vi "Main.vi"(11 "Module Admin":refnum<class "Delacor_lib_QMH_Module Admin.lvclass">) -> ()   [LabVIEW 2019, in "Acquisition.lvlib"]
doc: "This template is based off of the Queued Message Handler design pattern and the Queued Message Handler project template that ships with LabVIEW.\n\nThe main difference is that the queue is private to this module and communication between modules is performed via Broadcast and Request events.\n\nRequest events are wrapped in public API methods and are handled in the Event Handling Loop (EHL) of this VI. Any module can register for Broadcast events sent by this module. The EHL generates messages based on user interface actions.\n\nThe Message Handling Loop (MHL) processes messages generated by the EHL, or by other messages. The messages are string values, so new messages can be added easily to the Message Cases case structure in the MHL. Each message cluster can also provide an optional value for Message Data, which is a variant that can be converted to whatever message-specific data is required.\n_____\nBased on Delacor QMH Project Template 5.0.0.82."
uses:
  Acquisition.lvlib
  <vilib>/Delacor/Delacor QMH/Libraries/Module Admin_class/Delacor_lib_QMH_Module Admin.lvclass
  Module Data--cluster.ctl
  Stop Helper Loop Argument--cluster.ctl
  Stop Argument--cluster.ctl
  <vilib>/Delacor/Delacor QMH/Libraries/Message Queue_class/Delacor_lib_QMH_Message Queue.lvclass/Delacor_lib_QMH_Message Queue.ctl
  <vilib>/Delacor/Delacor QMH/Libraries/Module Admin_class/Delacor_lib_QMH_Module Admin.lvclass/Delacor_lib_QMH_Module Admin.ctl
  Start Aquire Argument--cluster.ctl
  Stop Acquire Argument--cluster.ctl
  <vilib>/Utility/miscctls.llb/LVPointTypeDef.ctl
  <vilib>/Delacor/Delacor QMH/Libraries/Message Queue_class/Delacor_lib_QMH_Enqueue Message (Single).vi
  <vilib>/Delacor/Delacor QMH/Libraries/Module Admin_class/Delacor_lib_QMH_Get External Launch.vi
  <vilib>/Utility/error.llb/Error Cluster From Error Code.vi
  <vilib>/ErrorRing/Error Ring.xnode
  <vilib>/Delacor/Delacor QMH/Libraries/Message Queue_class/Delacor_lib_QMH_Message Queue.lvclass
panel:
  out "Waveform Graph - Dark":dynamicdata(graph)
  out "error out":errorcluster
  out "Status":string
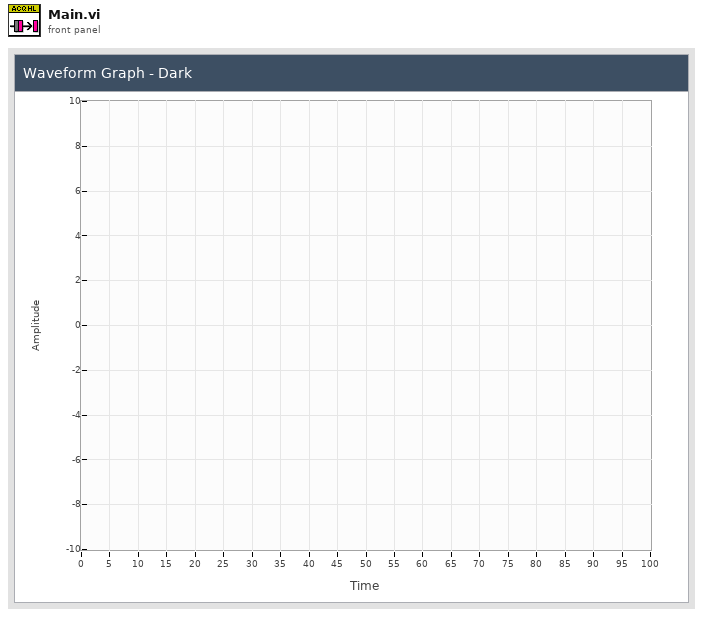
[diagram p1: front panel]
types:
  T1 = typedef "Acquisition.lvlib/Request Events--cluster.ctl" = cluster{"Stop Module":refnum<user-event>, "Show Panel":refnum<user-event>, "Hide Panel":refnum<user-event>, "Get Module Execution Status":refnum<user-event>, "Show Diagram":refnum<user-event>, "Start Helper Loop":refnum<user-event>, "Stop Helper Loop":refnum<user-event>, "Start Aquire":refnum<user-event>, "Stop Acquire":refnum<user-event>}
  T2 = typedef "Acquisition.lvlib/Module Data--cluster.ctl" = cluster{"Status":string}
  T3 = typedef "Acquisition.lvlib/Stop Helper Loop Argument--cluster.ctl" = cluster{"Boolean":bool}
  T4 = enum32{"invalid lock state", "Not Locked", "Locked (No Password)", "Password-protected"}
  T5 = typedef "Acquisition.lvlib/Stop Argument--cluster.ctl" = cluster{"Origin":string, "Exit via Stop Module Req?":bool, "Wait for Module to stop?":bool}
  T6 = typedef "Acquisition.lvlib/Start Aquire Argument--cluster.ctl" = cluster{"Boolean":bool}
  T7 = typedef "Acquisition.lvlib/Stop Acquire Argument--cluster.ctl" = cluster{"Boolean":bool}
  T8 = typedef "LVPointTypeDef.ctl" = cluster{"Horizontal":i16, "Vertical":i16}
  T9 = enum32{"Invalid", "Standard", "Closed", "Hidden", "Minimized", "Maximized"}
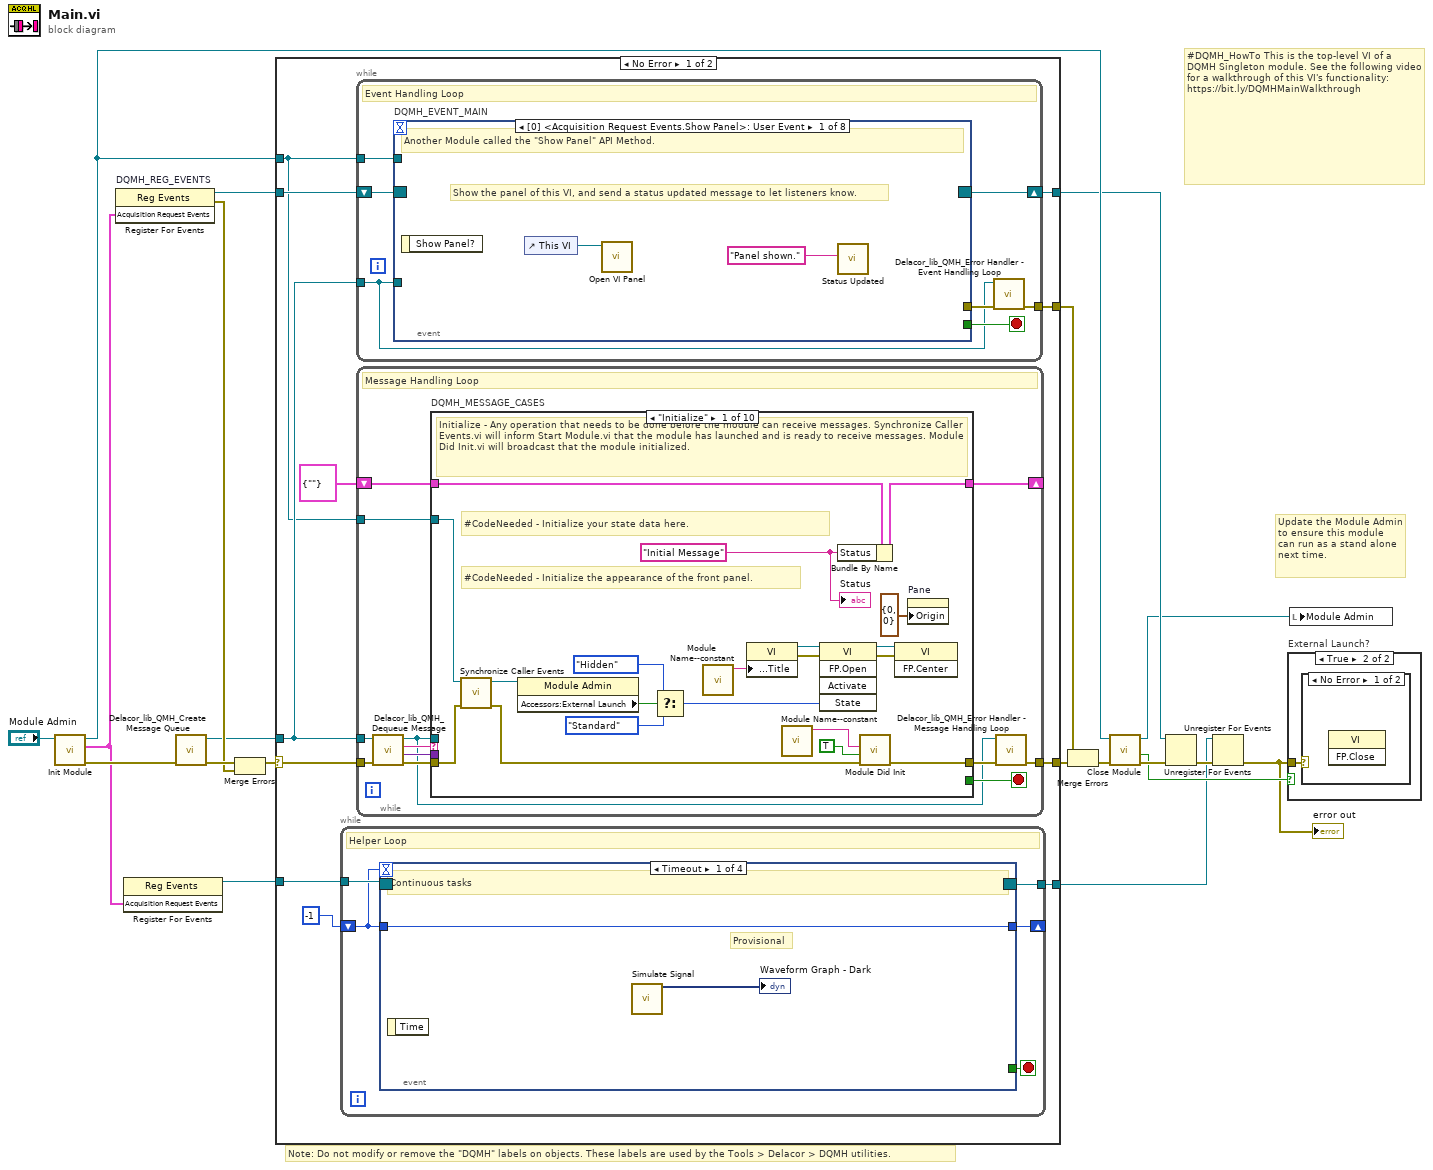
[diagram p0: block diagram]
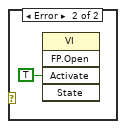
[diagram p3: hidden frame]
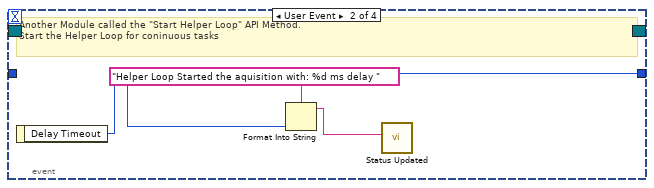
[diagram p4: hidden frame]
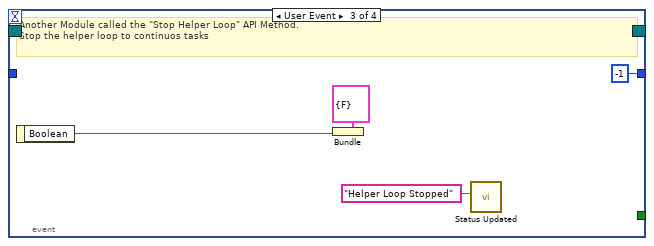
[diagram p5: hidden frame]
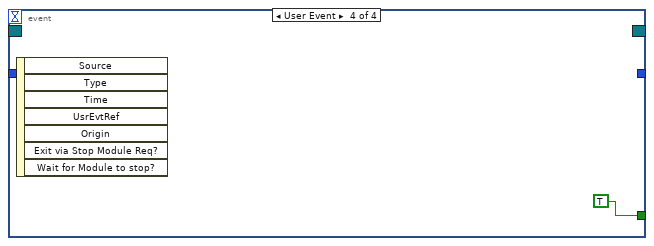
[diagram p6: hidden frame]
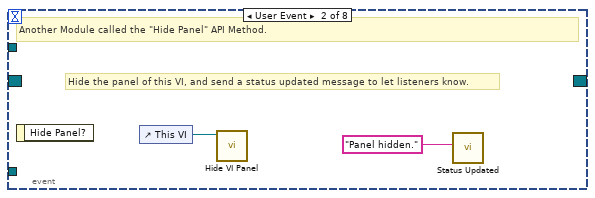
[diagram p7: hidden frame]
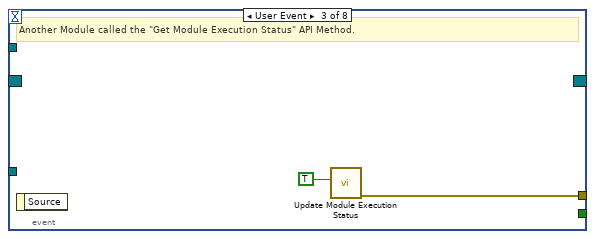
[diagram p8: hidden frame]
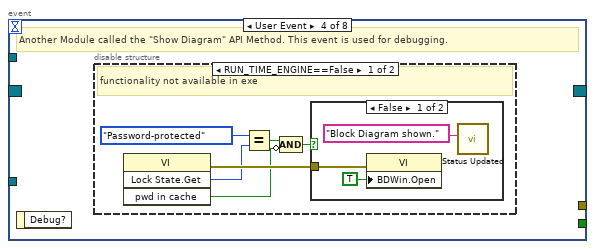
[diagram p9: hidden frame]
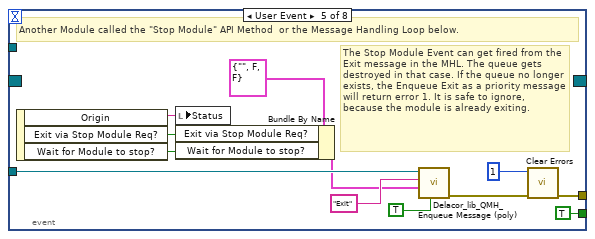
[diagram p12: hidden frame]
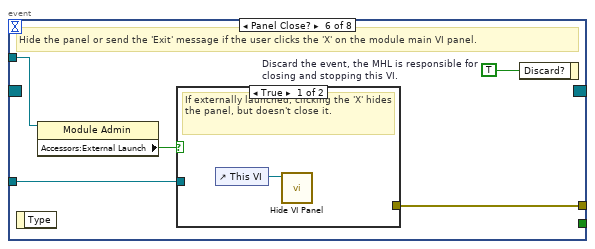
[diagram p13: hidden frame]
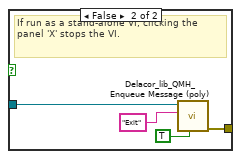
[diagram p14: hidden frame]
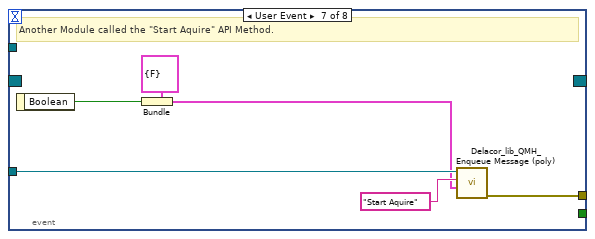
[diagram p15: hidden frame]
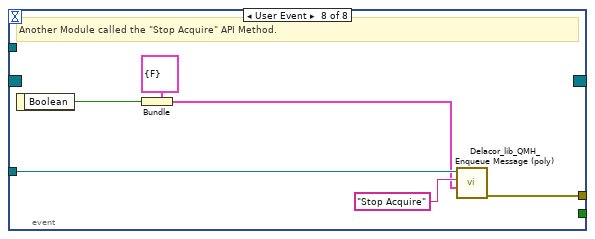
[diagram p16: hidden frame]
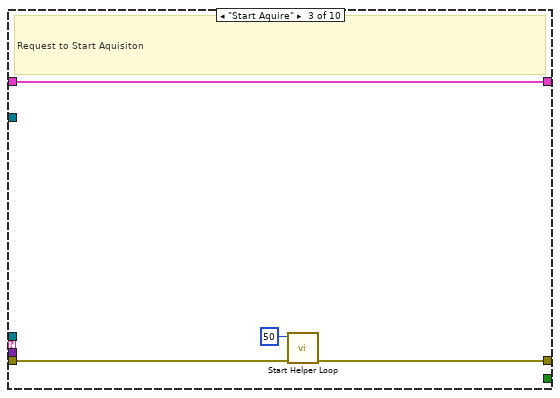
[diagram p18: hidden frame]
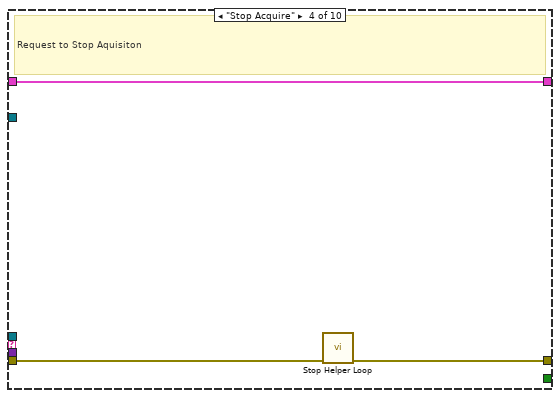
[diagram p19: hidden frame]
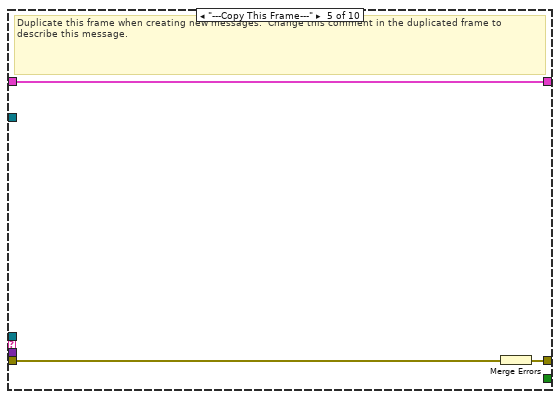
[diagram p20: hidden frame]
diagram:
  # "#DQMH_HowTo This is the top-level VI of a DQMH Singleton module. See the following video for a walkthrough of this VI's functionality: https://bit.ly/DQMHMainWalkthrough"
  # "Note: Do not modify or remove the \"DQMH\" labels on objects. These labels are used by the Tools > Delacor > DQMH utilities."
  # "Update the Module Admin to ensure this module can run as a stand alone next time."
  n1 = call "Init Module.vi"("Singleton Module Admin in"="Module Admin") -> ("error out"=w19:errorcluster, "Acquisition Request Events"=w4:T1, "Singleton Module Admin out"=w12:refnum<class "Delacor_lib_QMH_Module Admin.lvclass">)  [unwired: 8 in]
  n2 = register-events "DQMH_REG_EVENTS"(w4) -> (reference out=w10:refnum<event-registration>, error out=w13:errorcluster)  [unwired: 2 in]
  n3 = register-events(w4) -> (reference out=w5:refnum<event-registration>)  [unwired: 2 in, 1 out]
  n4 = call <vilib>:"Delacor_lib_QMH_Create Message Queue.vi"("error in (no error)"=w19) -> ("error out"=w15:errorcluster, "Message Queue"=w9:refnum<class "Delacor_lib_QMH_Message Queue.lvclass">)  [unwired: 9 in]
  n5 = Merge Errors(w15, w13) -> (w14:errorcluster)
  n6 = case shown="No Error" w14 {
    selector: w14 -> [w29 w210]
    tunnel: [w31 w209] -> w20
    tunnel: [w28 w215] -> w11
    tunnel: w10 -> [w26 w215]
    tunnel: w9 -> [w25 w208]
    tunnel: [w30 _] -> w17
    tunnel: w12 -> [w24 w211]
    tunnel: w5 -> [w23 w207]
    tunnel: [w22 w207] -> w1
    frame No Error {
      n7 = while {
        tunnel: w23 -> [w36]
        tunnel: [w35] -> w22
        shift-right: [w33] -> _
        shift-left: -1 -> [w32]
        stop <- w34 stop-if-true
        # "Helper Loop"
        n8 = event shown="[0] Timeout" {
          selector: w36 -> [_ _ _ _]
          dyn-events: [_ _ _ _] -> w35
          timeout: w32 -> [_ _ _ _]
          tunnel: [_ _ _ TRUE] -> w34
          tunnel: [w38 w41 -1 _] -> w33
          tunnel: w32 -> [w38 _ _ _]
          event Timeout {
            # "Provisional"
            # "Continuous tasks"
            n9 = event-data() -> ()  [unwired: 1 in, 1 out]
            n10 = call "Simulate Signal"() -> ("Sine"=→"Waveform Graph - Dark":dynamicdata)  [unwired: 14 in, 1 out]
          }
          event User Event {
            # "Another Module called the \"Start Helper Loop\" API Method.\nStart the Helper Loop for coninuous tasks"
            n11 = event-data() -> ("Delay Timeout"=w41:u32)  [unwired: 1 in]
            n12 = Format Into String(format string="Helper Loop Started the aquisition with: %d ms delay ", w41) -> (resulting string=w40:string)  [unwired: 2 in, 1 out]
            n13 = call "Status Updated.vi"("Status"=w40) -> ()  [unwired: 10 in, 1 out]
          }
          event User Event {
            # "Another Module called the \"Stop Helper Loop\" API Method.\nStop the helper loop to continuos tasks"
            n14 = event-data() -> ("Boolean"=w44:bool)  [unwired: 1 in]
            n15 = Bundle(cluster=T3 {"Boolean"=FALSE} ("Stop Helper Loop Argument"), "Boolean"=w44) -> ()  [unwired: 1 out]
            n16 = call "Status Updated.vi"("Status"="Helper Loop Stopped") -> ()  [unwired: 10 in, 1 out]
          }
          event User Event {
            n17 = event-data() -> ()  [unwired: 1 in, 7 out]
          }
        }
      }
      n18 = while {
        tunnel: w25 -> [w47]
        shift-right: [w50] -> w28
        shift-left: w26 -> [w51]
        tunnel: [w52] -> w30
        tunnel: w24 -> [w48]
        stop <- w49 stop-if-true
        # "Event Handling Loop"
        n19 = event "DQMH_EVENT_MAIN" shown="[0] <Acquisition Request Events.Show Panel>: User Event" {
          selector: w51 -> [_ _ _ _ _ _ _ _]
          dyn-events: [_ _ _ _ _ _ _ _] -> w50
          timeout: _ -> [_ _ _ _ _ _ _ _]
          tunnel: [_ _ _ _ TRUE ("Discard?") _ _ _] -> w49
          tunnel: w47 -> [_ _ _ _ w76 w83 w96 w102]
          tunnel: [_ _ w59 _ w79 w85 w91 w97] -> w53
          tunnel: w48 -> [_ _ _ _ _ w82 _ _]
          event User Event {
            # "Show the panel of this VI, and send a status updated message to let listeners know."
            # "Another Module called the \"Show Panel\" API Method."
            n20 = event-data() -> ()  [unwired: 1 in, 1 out]
            n21 = control-ref of="This VI"() -> (w55:refnum<vi>)
            n22 = call "Open VI Panel.vi"("VI"=w55) -> ()  [unwired: 10 in, 1 out]
            n23 = call "Status Updated.vi"("Status"="Panel shown." ("format string")) -> ()  [unwired: 10 in, 1 out]
          }
          event User Event {
            # "Hide the panel of this VI, and send a status updated message to let listeners know."
            # "Another Module called the \"Hide Panel\" API Method."
            n24 = event-data() -> ()  [unwired: 1 in, 1 out]
            n25 = control-ref of="This VI"() -> (w57:refnum<vi>)
            n26 = call "Hide VI Panel.vi"("VI"=w57) -> ()  [unwired: 10 in, 1 out]
            n27 = call "Status Updated.vi"("Status"="Panel hidden." ("format string")) -> ()  [unwired: 10 in, 1 out]
          }
          event User Event {
            # "Another Module called the \"Get Module Execution Status\" API Method."
            n28 = event-data() -> ()  [unwired: 1 in, 1 out]
            n29 = call "Update Module Execution Status.vi"("Running?"=TRUE) -> ("error out"=w59:errorcluster)  [unwired: 10 in]
          }
          event User Event {
            # "Another Module called the \"Show Diagram\" API Method. This event is used for debugging."
            n30 = event-data() -> ()  [unwired: 1 in, 1 out]
            n31 = disable-structure shown="RUN_TIME_ENGINE==False" {
              frame condition #0 (active) {
                # "functionality not available in exe"
                n32 = invoke class="VI" method="Lock State.Get"() -> (error out=w65:errorcluster, "Get Lock State"=w64:T4, "pwd in cache"=w61:bool)  [unwired: 4 in, 1 out]
                n33 = Equal?(x=T4."Password-protected", y=w64) -> (x = y?=w62:bool)
                n34 = Compound Arithmetic op=AND(w62, invert w61) -> (w60:bool)
                n35 = case shown="False" w60 {
                  tunnel: w65 -> [w68 _]
                  frame False {
                    n36 = property class="VI"(error in=w68, "BDWin.Open"=TRUE ("Block Diagram Window:Open")) -> ()  [unwired: 1 in, 2 out]
                    n37 = call "Status Updated.vi"("Status"="Block Diagram shown." ("format string")) -> ()  [unwired: 10 in, 1 out]
                  }
                  frame True {
                    # "Password-protected VI, and the password is not in the cache. Do not show the diagram."
                  }
                }
              }
              frame condition #1 {
              }
            }
          }
          event User Event {
            # "The Stop Module Event can get fired from the Exit message in the MHL. The queue gets destroyed in that case. If the queue no longer exists, the Enqueue Exit as a priority message will return error 1. It is safe to ignore, because the module is already exiting."
            # "Another Module called the \"Stop Module\" API Method  or the Message Handling Loop below."
            n38 = event-data() -> ("Origin"=w75:string, "Exit via Stop Module Req?"=w71:bool, "Wait for Module to stop?"=w70:bool)  [unwired: 1 in]
            n39 = local write "Status"(w75) -> ()
            n40 = Bundle By Name(cluster=T5 {"Origin"="", "Exit via Stop Module Req?"=FALSE, "Wait for Module to stop?"=FALSE} ("Stop Argument"), "Exit via Stop Module Req?"=w71, "Wait for Module to stop?"=w70) -> (w69:T5)
            n41 = call-poly <vilib>:"Delacor_lib_QMH_Enqueue Message (poly).vi"("Priority Message? (F)"=TRUE, "Message Data"=w69, "Message"="Exit", "Message Queue in"=w76) -> ("error out"=w80:errorcluster)  [unwired: 6 in, 1 out]
            n42 = call <vilib>:"Clear Errors.vi"("error in (no error)"=w80, "specific error code to clear (0: all)"=1) -> ("error out"=w79:errorcluster)  [unwired: 4 in, 1 out]
          }
          event Panel Close? {
            w84 = TRUE  # Discard the event, the MHL is responsible for closing and stopping this VI.
            # "Hide the panel or send the 'Exit' message if the user clicks the 'X' on the module main VI panel."
            n43 = event-data() -> ()  [unwired: 1 in, 1 out]
            n44 = property class="Module Admin"(reference=w82) -> ("Accessors:External Launch"=w81:bool)  [unwired: 1 in, 2 out]
            n45 = case shown="True" w81 {
              tunnel: w83 -> [_ w89]
              tunnel: [_ w90] -> w85
              frame True {
                # "If externally launched, clicking the 'X' hides the panel, but doesn't close it."
                n46 = control-ref of="This VI"() -> (w86:refnum<vi>)
                n47 = call "Hide VI Panel.vi"("VI"=w86) -> ()  [unwired: 10 in, 1 out]
              }
              frame False {
                # "If run as a stand-alone VI, clicking the panel 'X' stops the VI."
                n48 = call-poly <vilib>:"Delacor_lib_QMH_Enqueue Message (poly).vi"("Priority Message? (F)"=TRUE, "Message"="Exit", "Message Queue in"=w89) -> ("error out"=w90:errorcluster)  [unwired: 7 in, 1 out]
              }
            }
            n49 = event-data("Discard?"=w84) -> ()  [unwired: 1 in, 1 out]
          }
          event User Event {
            # "Another Module called the \"Start Aquire\" API Method."
            n50 = event-data() -> ("Boolean"=w92:bool)  [unwired: 1 in]
            n51 = Bundle(cluster=T6 {"Boolean"=FALSE} ("Start Aquire Argument"), "Boolean"=w92) -> (w93:T6)
            n52 = call-poly <vilib>:"Delacor_lib_QMH_Enqueue Message (poly).vi"("Message Data"=w93, "Message"="Start Aquire", "Message Queue in"=w96) -> ("error out"=w91:errorcluster)  [unwired: 7 in, 1 out]
          }
          event User Event {
            # "Another Module called the \"Stop Acquire\" API Method."
            n53 = event-data() -> ("Boolean"=w98:bool)  [unwired: 1 in]
            n54 = Bundle(cluster=T7 {"Boolean"=FALSE} ("Stop Acquire Argument"), "Boolean"=w98) -> (w99:T7)
            n55 = call-poly <vilib>:"Delacor_lib_QMH_Enqueue Message (poly).vi"("Message Data"=w99, "Message"="Stop Acquire", "Message Queue in"=w102) -> ("error out"=w97:errorcluster)  [unwired: 7 in, 1 out]
          }
        }
        n56 = call-dynamic "Delacor_lib_QMH_Error Handler - Event Handling Loop.vi"("error in (no error)"=w53, "Message Queue in"=w47) -> ("dup error in"=w52:errorcluster)  [unwired: 8 in, 1 out]
      }
      n57 = while {
        tunnel: w25 -> [w105]
        shift-right: [w109] -> _
        shift-left: T2 {"Status"=""} ("Data Cluster") -> [w110]
        tunnel: w29 -> [w113]
        tunnel: [w111] -> w31
        tunnel: w24 -> [w103]
        stop <- w108 stop-if-true
        # "Message Handling Loop"
        n58 = call-dynamic "Delacor_lib_QMH_Dequeue Message.vi"("error in (no error)"=w113, "Message Queue in"=w105) -> ("error out"=w112:errorcluster, "Message Data"=w106:variant, "Message"=w107:string, "Message Queue out"=w104:refnum<class "Delacor_lib_QMH_Message Queue.lvclass">)  [unwired: 6 in]
        n59 = case "DQMH_MESSAGE_CASES" shown="\"Initialize\"" w107 {
          selector: w107 -> [_ _ _ _ _ _ _ _ _ w194]
          tunnel: w104 -> [_ _ _ _ _ _ _ w164 w186 _]
          tunnel: w112 -> [w132 w136 w139 w142 w146 w148 w153 w171 w192 w196]
          tunnel: [w130 w136 w138 w141 w145 w148 w152 w167 w189 w197] -> w114
          tunnel: w110 -> [w121 w135 w140 w143 w144 w147 w150 w166 w185 w195]
          tunnel: [w120 w135 w140 w143 w144 w147 w150 w166 w185 w195] -> w109
          tunnel: [_ _ _ _ _ _ _ _ w184 _] -> w108
          tunnel: w106 -> [_ _ _ _ _ _ _ w165 w183 _]
          tunnel: w103 -> [w122 _ _ _ _ _ _ w163 w178 _]
          frame "Initialize" {
            w115 = "Initial Message" ("Initial Message")
            # "#CodeNeeded - Initialize the appearance of the front panel."
            # "#CodeNeeded - Initialize your state data here."
            # "Initialize - Any operation that needs to be done before the module can receive messages. Synchronize Caller Events.vi will inform Start Module.vi that the module has launched and is ready to receive messages. Module Did Init.vi will broadcast that the module initialized."
            n60 = call "Synchronize Caller Events.vi"("error in (no error)"=w132, "Singleton Module Admin in"=w122) -> ("error out"=w131:errorcluster, "Singleton Module Admin out"=w117:refnum<class "Delacor_lib_QMH_Module Admin.lvclass">)  [unwired: 8 in]
            n61 = property class="Module Admin"(reference=w117) -> ("Accessors:External Launch"=w126:bool)  [unwired: 1 in, 2 out]
            n62 = Select(t=T9."Hidden" ("State"), s=w126, f=T9."Standard" ("State")) -> (s? t:f=w123:T9)
            n63 = call "Module Name--constant.vi"() -> ("Module Name"=w129:string)  [unwired: 11 in]
            n64 = property class="VI"("Front Panel.Title"=w129) -> (reference out=w128:refnum<vi>, error out=w134:errorcluster)  [unwired: 2 in]
            n65 = call "Module Name--constant.vi"() -> ("Module Name"=w118:string)  [unwired: 11 in]
            n66 = invoke class="VI" method="FP.Open"(reference=w128, error in=w134, "State"=w123) -> (reference out=w127:refnum<vi>, error out=w133:errorcluster)  [unwired: 2 in, 3 out]
            n67 = Bundle By Name(cluster=w121, "Status"=w115) -> (w120:T2)
            n68 = call "Module Did Init.vi"("error in (no error)"=w131, "Initialized?"=TRUE, "Origin"=w118) -> ("error out"=w130:errorcluster)  [unwired: 8 in]
            n69 = invoke class="VI" method="FP.Center"(reference=w127, error in=w133) -> ()  [unwired: 1 in, 3 out]
            n70 = property on="Pane" class="Pane"("Origin"=T8 {"Horizontal"=0, "Vertical"=0}) -> ()  [unwired: 2 in, 2 out]
            "Status" <- w115
          }
          frame "--- Module Specific ---" {
            # "Separator -- The following cases handle messages specific to this Module."
          }
          frame "Start Aquire" {
            # "Request to Start Aquisiton"
            n71 = call "Start Helper Loop.vi"("error in (no error)"=w139, "Delay Timeout"=u32 50) -> ("error out"=w138:errorcluster)  [unwired: 9 in]
          }
          frame "Stop Acquire" {
            # "Request to Stop Aquisiton"
            n72 = call "Stop Helper Loop.vi"("error in (no error)"=w142) -> ("error out"=w141:errorcluster)  [unwired: 10 in]
          }
          frame "---Copy This Frame---" {
            # "Duplicate this frame when creating new messages.  Change this comment in the duplicated frame to describe this message."
            n73 = Merge Errors(w146) -> (w145:errorcluster)
          }
          frame "--- Exit and Error Handling---" {
            # "Separator - The following cases handle errors and exit messages."
          }
          frame "Simulate MHL Error" {
            # "#DQMH_HowTo The 'Simulate MHL Error' button  illustrates how the MHL handles errors. This event is instructional in nature and can be removed."
            # "Simulate an error occurring at the MHL"
            n74 = call "Module Name--constant.vi"() -> ("Module Name"=w149:string)  [unwired: 11 in]
            n75 = xnode "Error Ring"("parameter 0"=w149) -> ("error out"=w151:errorcluster)
            n76 = Merge Errors(w153, w151) -> (w152:errorcluster)
          }
          frame "Error" {
            # "#CodeRecommended - If you ever change the name of this \"Error\" message, you'll need to update the name in the Check Loop Error.vi as well."
            # "#CodeRecommended - If the module is running in standalone mode (External Launch = FALSE), this code will pop up an error dialog and call the 'Exit' message if an error occurs. Add more fine-grained error handling here."
            # "Error - Check the error message data and respond accordingly. This message is sent by the \"Error Handler\" VIs at the end of each loop in this application."
            n77 = property class="Module Admin"(reference=w163) -> ("Accessors:External Launch"=w162:bool)  [unwired: 1 in, 2 out]
            n78 = Variant To Data(error in=w171, type=errorcluster {"status"=FALSE, "code"=0, "source"=""} ("error constant"), Variant=w165) -> (data=w172:errorcluster, error out=w169:errorcluster)
            n79 = call "Module Name--constant.vi"() -> ("Module Name"=w161:string)  [unwired: 11 in]
            n80 = call "Error Reported.vi"("Additional Information"=w161, "Error"=w172) -> ()  [unwired: 9 in, 1 out]
            n81 = case shown="False" w162 {
              tunnel: [w177 _] -> w168
              tunnel: w164 -> [w175 _]
              tunnel: w172 -> [w176 _]
              frame False {
                # "If the module is running standalone, then pop up an error dialog and call the \"Exit\" message."
                n82 = call <vilib>:"Simple Error Handler.vi"("error in (no error)"=w176) -> ()  [unwired: 4 in, 5 out]
                n83 = call-poly <vilib>:"Delacor_lib_QMH_Enqueue Message (poly).vi"("Priority Message? (F)"=TRUE, "Message"="Exit", "Message Queue in"=w175) -> ("error out"=w177:errorcluster)  [unwired: 7 in, 1 out]
              }
              frame True {
                # "If the module was launched externally, calling the Error Reported broadcast VI is the only action performed by the \"Error\" message. The module's caller can then process the error appropriately."
              }
            }
            n84 = Merge Errors(w169, w168) -> (w167:errorcluster)
            n85 = local write "error out"(w167) -> ()
          }
          frame "Exit" {
            w182 = 91  # 91: not all Exit messages will have an argument
            w184 = TRUE  # Stop the VI
            # "Release the message queue reference"
            # "#CodeNeeded - Add any required cleanup code here"
            # "Exit - Exit the application."
            n86 = Variant To Data(error in=w192, type=T5 {"Origin"="", "Exit via Stop Module Req?"=FALSE, "Wait for Module to stop?"=FALSE} ("Stop Argument"), Variant=w183) -> (data=w180:T5, error out=w188:errorcluster)
            n87 = call <vilib>:"Clear Errors.vi"("error in (no error)"=w188, "specific error code to clear (0: all)"=w182) -> ("error out"=w191:errorcluster)  [unwired: 4 in, 1 out]
            n88 = control-ref of="This VI"() -> (w179:refnum<vi>)
            n89 = call-dynamic "Delacor_lib_QMH_Release Message Queue.vi"("error in (no error)"=w191, "Message Queue"=w186) -> ("error out"=w190:errorcluster)  [unwired: 9 in]
            n90 = call "Handle Exit.vi"("Stop Argument"=w180, "Admin in"=w178, "VI reference"=w179) -> ("error out"=w187:errorcluster)  [unwired: 7 in, 1 out]
            n91 = Merge Errors(w190, w187) -> (w189:errorcluster)
          }
          frame Default {
            # "'Default' case only runs if there is a message that isn't defined in any of the other cases.  Output a programming error."
            n92 = call "Module Name--constant.vi"() -> ("Module Name"=w193:string)  [unwired: 11 in]
            n93 = xnode "Error Ring"("parameter 0"=w194, "parameter 1"=w193) -> ("error out"=w198:errorcluster)
            n94 = Merge Errors(w196, w198) -> (w197:errorcluster)
          }
        }
        n95 = call-dynamic "Delacor_lib_QMH_Error Handler - Message Handling Loop.vi"("error in (no error)"=w114, "Message Queue in"=w104) -> ("dup error in"=w111:errorcluster)  [unwired: 8 in, 1 out]
      }
    }
    frame Error {
      # "Synchronize Caller Events.vi will inform Start Module.vi that the module has launched and will let the code calling Start Module.vi register for broadcasts and would permit the caller receive the broadcast that an error occurred at launch time."
      n96 = call-dynamic "Delacor_lib_QMH_Release Message Queue.vi"("error in (no error)"=w210, "Message Queue"=w208) -> ("error out"=w209:errorcluster)  [unwired: 9 in]
      n97 = call "Synchronize Caller Events.vi"("Singleton Module Admin in"=w211) -> ("error out"=w216:errorcluster)  [unwired: 9 in, 1 out]
      n98 = call "Module Name--constant.vi"() -> ("Module Name"=w214:string)  [unwired: 11 in]
      n99 = Format Into String(format string="An error occurred during initialization. %s is no longer running.", w214) -> (resulting string=w212:string)  [unwired: 2 in, 1 out]
      n100 = Merge Errors(w209, w216) -> (w217:errorcluster)
      n101 = call "Error Reported.vi"("Additional Information"=w212, "Error"=w217) -> ()  [unwired: 9 in, 1 out]
    }
  }
  n102 = Merge Errors(w17, w20) -> (w16:errorcluster)
  n103 = call "Close Module.vi"("error in (no error)"=w16, "Module Admin in"=w12) -> ("error out"=w18:errorcluster, "External Launch"=w6:bool, "Module Admin out"=w7:refnum<class "Delacor_lib_QMH_Module Admin.lvclass">)  [unwired: 7 in]
  n104 = Unregister For Events(event registration refnum=w11, error in=w18) -> (error out=w3:errorcluster)
  n105 = Unregister For Events(event registration refnum=w1, error in=w3) -> (error out=w2:errorcluster)
  "error out" <- w2
  n106 = case "External Launch?" shown="True" w6 {
    tunnel: w2 -> [_ w218]
    frame False {
    }
    frame True {
      n107 = case shown="No Error" w218 {
        frame No Error {
          n108 = invoke class="VI" method="FP.Close"() -> ()  [unwired: 3 in, 3 out]
        }
        frame Error {
          n109 = invoke class="VI" method="FP.Open"("Activate"=TRUE ("Activate?")) -> ()  [unwired: 4 in, 5 out]
        }
      }
    }
  }
  n110 = local write "Module Admin"(w7) -> ()
